vi "Create Dataset 1D Integer.vi"(8 "Chunk size":u64, 9 "Dataset name":string, 10 "loc_id":i32, 11 "error in (no error)":errorcluster) -> (0 "Error code":i32, 2 "dataset_id":i32, 3 "error out":errorcluster)   [LabVIEW 2010]
uses:
  Release/HDF5Tools.dll
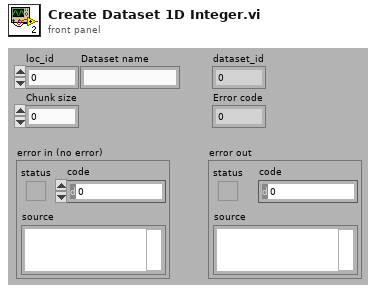
[diagram p1: front panel]
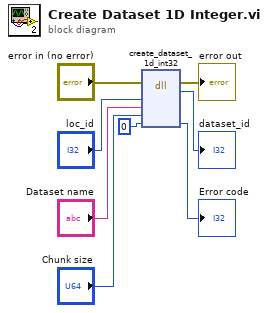
[diagram p0: block diagram]
diagram:
  n1 = dll-call lib="Z:/users/alex/projects/HDF5Tools/Release/HDF5Tools.dll" fn="create_dataset_1d_int32"(error in="error in (no error)", "loc_id"="loc_id", "name"="Dataset name", "chunk"="Chunk size", "error"=0) -> (error out=→"error out":errorcluster, "dataset_id"=→"dataset_id":i32, "error"=→"Error code":i32)  [unwired: 5 in, 1 out]
